vi "JSON to LVObject - Dictionary of Object with Array of Objects - Returns Object.vi"() -> ()   [LabVIEW 2017, in "Generic Object Serializer Tests.lvlib"]
uses:
  Generic Object Serializer Tests.lvlib
  Generic Object Serializer/Generic Object Serializer.lvclass
  Dictionary/Dictionary.lvclass
  <vilib>/addons/_JKI Toolkits/Caraya/classes/Assert/Assert Equal Value and Type_Variant.vi
  <vilib>/addons/_JKI Toolkits/Caraya/classes/Test/Test.lvclass
  <vilib>/addons/_JKI Toolkits/Caraya/classes/Assert/Assert.lvclass
panel:
  out "error out":errorcluster
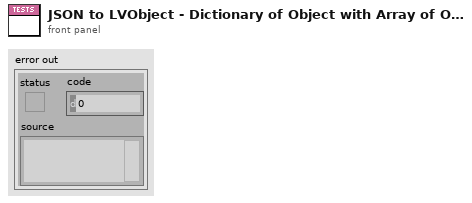
[diagram p1: front panel]
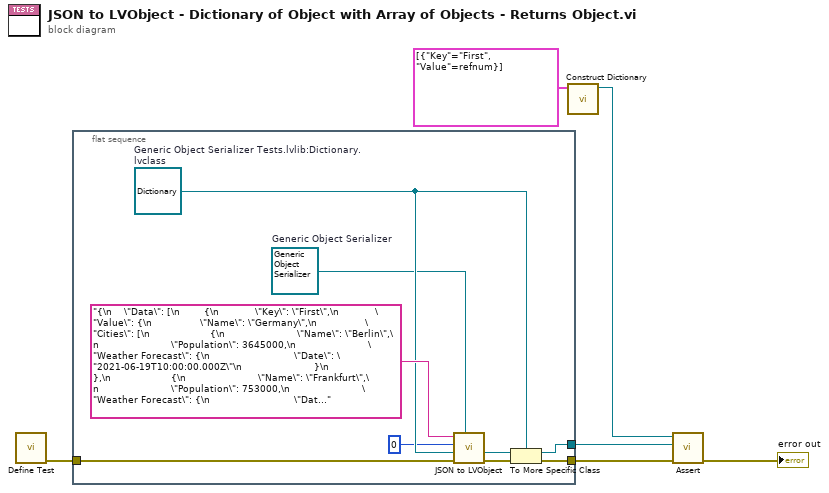
[diagram p0: block diagram]
diagram:
  n1 = call <vilib>:"Define Test.vi"() -> ("error out"=w6:errorcluster)  [unwired: 11 in]
  n2 = flat-sequence {
    tunnel: w6 -> [w9]
    tunnel: [w8] -> w4
    tunnel: [w7] -> w3
    frame #0 {
      w12 = refnum<class "Dictionary.lvclass"> refnum  # Generic Object Serializer Tests.lvlib:Dictionary.lvclass
      w10 = refnum<class "Generic Object Serializer.lvclass"> refnum  # Generic Object Serializer
      n3 = call-dynamic "JSON to LVObject.vi"("LVClass Serializer"=w10, "error in (no error)"=w9, "Object Type"=w12, "Offset"=0, "JSON"="{\n    \"Data\": [\n        {\n            \"Key\": \"First\",\n            \"Value\": {\n                \"Name\": \"Germany\",\n                \"Cities\": [\n                    {\n                        \"Name\": \"Berlin\",\n                        \"Population\": 3645000,\n                        \"Weather Forecast\": {\n                            \"Date\": \"2021-06-19T10:00:00.000Z\"\n                        }\n                    },\n                    {\n                        \"Name\": \"Frankfurt\",\n                        \"Population\": 753000,\n                        \"Weather Forecast\": {\n                            \"Date\": \"2021-06-19T10:00:00.000Z\"\n                        }\n                    }\n                ]\n            }\n        }\n    ]\n}") -> ("error out"=w15:errorcluster, "Object"=w13:refnum<class>)  [unwired: 5 in]
      n4 = To More Specific Class(target class=w12, reference=w13, error in=w15) -> (specific class reference=w7:refnum<class "Dictionary.lvclass">, error out=w8:errorcluster)
    }
  }
  n5 = call "Construct Dictionary.vi"("Data"=cluster{"Key":string, "Value":refnum<class>}[] [{"Key"="First", "Value"=refnum}]) -> ("Dictionary"=w2:refnum<class "Dictionary.lvclass">)  [unwired: 9 in, 1 out]
  n6 = call-poly <vilib>:"Assert.vi"("error in (no error)"=w4, "Y"=w3, "X"=w2) -> ("error out"=→"error out":errorcluster)  [unwired: 8 in]
